vi "Page HTML.vi"(11 "WS Port":u16) -> (3 "Page HTML":string)   [LabVIEW 2020, in "LV Server.lvclass"]
uses:
  LV Server.lvclass
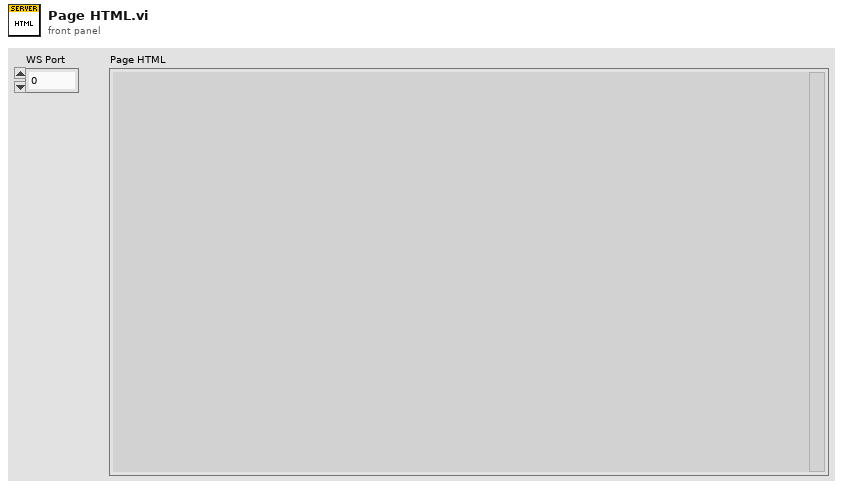
[diagram p1: front panel]
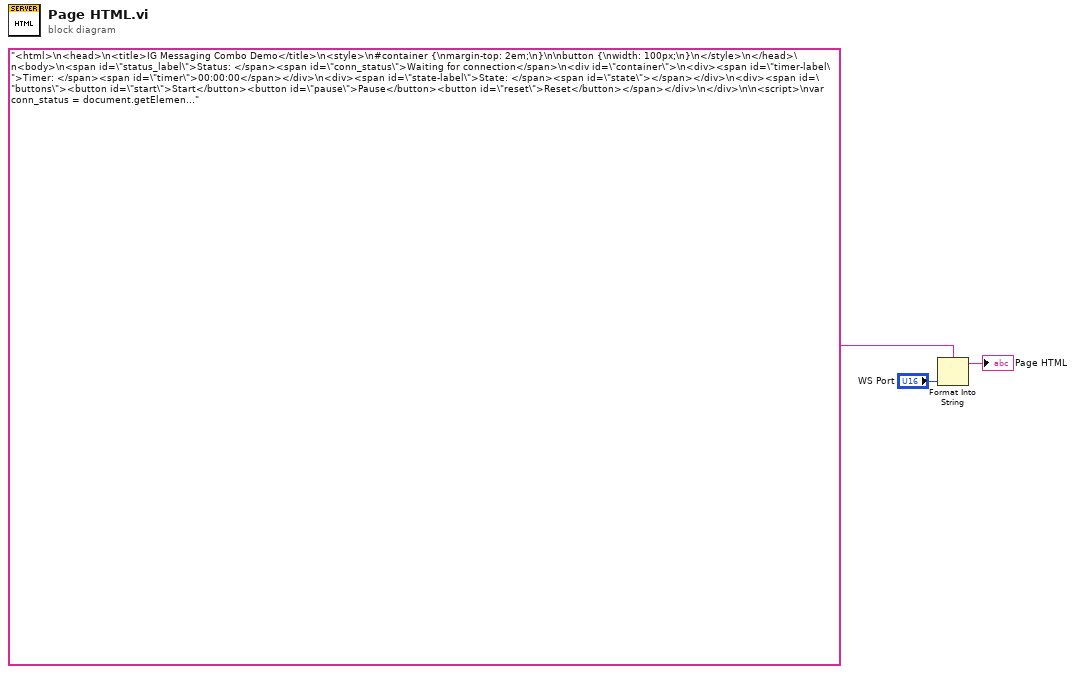
[diagram p0: block diagram]
diagram:
  n1 = Format Into String(format string="<html>\n<head>\n<title>IG Messaging Combo Demo</title>\n<style>\n#container {\nmargin-top: 2em;\n}\n\nbutton {\nwidth: 100px;\n}\n</style>\n</head>\n<body>\n<span id=\"status_label\">Status: </span><span id=\"conn_status\">Waiting for connection</span>\n<div id=\"container\">\n<div><span id=\"timer-label\">Timer: </span><span id=\"timer\">00:00:00</span></div>\n<div><span id=\"state-label\">State: </span><span id=\"state\"></span></div>\n<div><span id=\"buttons\"><button id=\"start\">Start</button><button id=\"pause\">Pause</button><button id=\"reset\">Reset</button></span></div>\n</div>\n\n<script>\nvar conn_status = document.getElementById(\"conn_status\");\nvar timer = document.getElementById(\"timer\");\nvar state = document.getElementById(\"state\");\n\nvar lvSock = new WebSocket(\"ws://127.0.0.1:%d/\");\n\nlvSock.onmessage = (event) => {\n\tvar msg = JSON.parse(event.data);\n\n\tswitch (msg.id) {\n\t\tcase 'Timer State':\n\t\t\tstate.innerText = msg.data;\n\t\t\tbreak;\n\n\t\tcase 'Timer Value':\n\t\t\ttimer.innerText = msg.data;\n\t\t\tbreak;\n\n\t\tcase 'Timer Init':\n\t\t\tstate.innerText = msg.data.State;\n\t\t\ttimer.innerText = msg.data.Value;\n\t\t\tbreak;\n\n\t\tdefault:\n\t\t\tconsole.log(\"Unknown msg.id: \" + msg.id);\n\t\t\tconsole.log(msg);\n\t}\n}\n\nlvSock.onopen = (event) => {\n\tconn_status.innerText = \"Connected\";\n\tconsole.log(\"Connected\");\n}\n\nlvSock.onerror = (event) => {\n\tconn_status.innerText = \"Error\";\n\tconsole.log(event);\n}\n\nlvSock.onclose = (event) => {\n\tconn_status.innerText = \"Disconnected\";\n\tconsole.log(\"Disconnected\");\n}\n\nfunction sendMsg(id, data) {\n\tvar msg = {id: id, data: data};\n\tconsole.log(msg);\n\tvar msgJSON = JSON.stringify(msg);\n\tconsole.log(msgJSON);\n\tlvSock.send(msgJSON);\n}\n\ndocument.getElementById(\"start\").onclick = (event) => {\n\tsendMsg(\"Timer Start\", true);\n}\n\ndocument.getElementById(\"pause\").onclick = (event) => {\n\tsendMsg(\"Timer Pause\", true);\n}\n\ndocument.getElementById(\"reset\").onclick = (event) => {\n\tsendMsg(\"Timer Reset\", true);\n}\n</script>\n</body>\n</html>", "WS Port") -> (resulting string=→"Page HTML":string)  [unwired: 2 in, 1 out]
